vi "GV line gating.vi"() -> ()   [LabVIEW 2017]
panel:
  in  "Line gating":bool
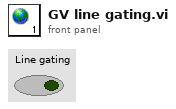
[diagram p1: front panel]
diagram:
